vi "Configure Trigger.vi"(6 "Manual Trigger Delay (1 s)":dbl=1.0, 7 "Trigger Level (0)":dbl, 8 "error in (no error)":errorcluster, 9 "Auto Delay (F:Disable)":bool, 10 "Trigger Source (0: Immediate)":i32(ring) items=["Immediate", "Software (Bus)", "External", "Internal"], 11 "VISA resource name":refnum<visa-resource-name>) -> (0 "error out":errorcluster, 3 "VISA resource name out":refnum<visa-resource-name>)   [LabVIEW 2020, in "Agilent 3446X Series.lvlib"]
doc: "Configures the trigger settings on the instrument.\n\n<B>Note:</B> Use this VI only with other low-level VIs. The high-level VIs automatically incorporate this functionality."
uses:
  <instrlib>/Agilent 3446X Series/Agilent 3446X Series.lvlib
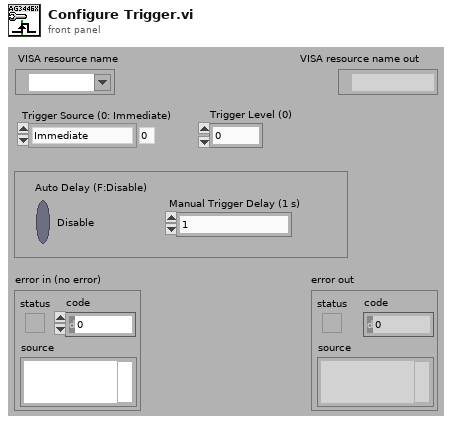
[diagram p1: front panel]
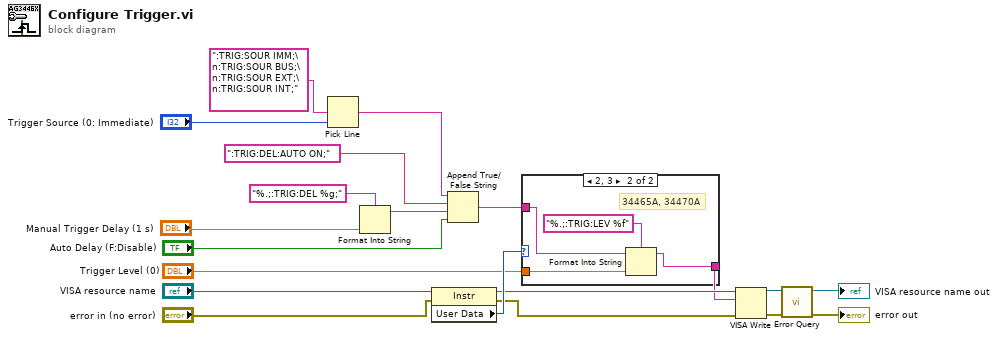
[diagram p0: block diagram]
diagram:
  n1 = Pick Line(multi-line string=":TRIG:SOUR IMM;\n:TRIG:SOUR BUS;\n:TRIG:SOUR EXT;\n:TRIG:SOUR INT;" ("Trigger Source"), line index="Trigger Source (0: Immediate)") -> (output string=w13:string)  [unwired: 1 out]
  n2 = Format Into String(format string="%.;:TRIG:DEL %g;" ("Manual Trigger Delay"), "Manual Trigger Delay (1 s)") -> (resulting string=w14:string)  [unwired: 2 in, 1 out]
  n3 = property class="Instr"(reference="VISA resource name", error in="error in (no error)") -> (reference out=w5:refnum<visa-resource-name>, error out=w4:errorcluster, "User Data"=w7:u32)
  n4 = Append True/False String(1:"Auto Delay (F:Disable)", 2:w14, 3:":TRIG:DEL:AUTO ON;" ("Enable Auto Delay"), 4:w13) -> (0:w8:string)
  n5 = case shown="2, 3" w7 {
    tunnel: w8 -> [w21 w23]
    tunnel: [w21 w24] -> w2
    tunnel: "Trigger Level (0)" -> [_ w25]
    frame 0, 4, Default {
      # "EDU34450A, 34460A, 34461A"
    }
    frame 2, 3 {
      # "34465A, 34470A"
      n6 = Format Into String(format string="%.;:TRIG:LEV %f", initial string=w23, w25) -> (resulting string=w24:string)  [unwired: 1 in, 1 out]
    }
  }
  n7 = VISA Write(VISA resource name=w5, write buffer=w2, error in (no error)=w4) -> (VISA resource name out=w12:refnum<visa-resource-name>, error out=w11:errorcluster)  [unwired: 1 out]
  n8 = call <instrlib>:"Error Query.vi"("error in (no error)"=w11, "VISA resource name"=w12) -> ("error out"=→"error out":errorcluster, "VISA resource name out"=→"VISA resource name out":refnum<visa-resource-name>)  [unwired: 8 out]
